vi "Draw Filled Rect.vi"(8 "Limits":dbl[](array[numeric]), 9 "Vision Instrumentation":T1, 10 "Target Data":T2={"Bounds"={"Left"=0.0, "Top"=0.0, "Right"=0.0, "Bottom"=0.0}, "Scores"={"Rect Coverage"=76.0, "Aspect Ratio"=0.0, "X Edge Strength"=40.0, "Y Edge Strength"=50.0}, "Clipped Edge"={"Left"=FALSE, "Top"=FALSE, "Right"=FALSE, "Bottom"=FALSE}}, 11 "image in":T3) -> (3 "image out":T3)   [LabVIEW 2011]
doc: "Add a rectangle border around the inside and outside of what is believed to be the reflective tape. Also place the color coded scores next to all of the large blobs being processed."
uses:
  <vilib>/vision/Image Controls.llb/IMAQ Image.ctl
  Target Data.ctl
  Vision Instrumentation Control.ctl
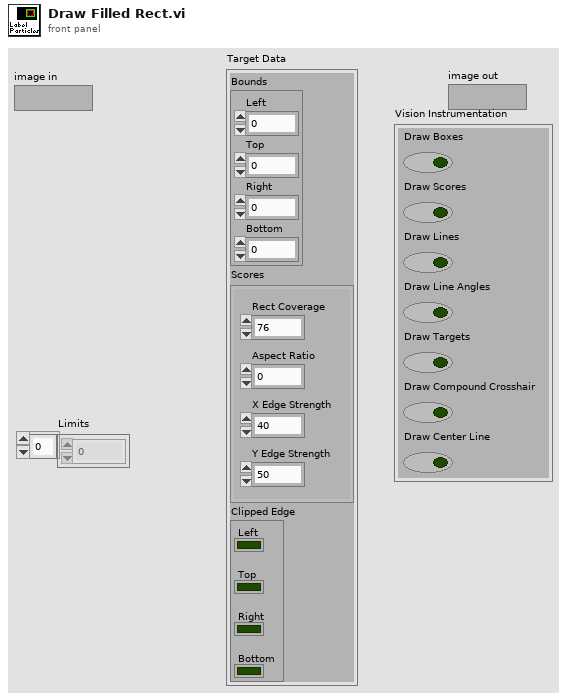
[diagram p1: front panel]
types:
  T1 = typedef "Vision Instrumentation Control.ctl" = cluster{"Draw Boxes":bool, "Draw Scores":bool, "Draw Lines":bool, "Draw Line Angles":bool, "Draw Targets":bool, "Draw Compound Crosshair":bool, "Draw Center Line":bool}
  T2 = typedef "Target Data.ctl" = cluster{"Bounds":cluster{"Left":dbl, "Top":dbl, "Right":dbl, "Bottom":dbl}, "Scores":cluster{"Rect Coverage":dbl, "Aspect Ratio":dbl, "X Edge Strength":dbl, "Y Edge Strength":dbl}, "Clipped Edge":cluster{"Left":bool, "Top":bool, "Right":bool, "Bottom":bool}}
  T3 = typedef "IMAQ Image.ctl" = refnum<image>
  T4 = cluster{"Left":dbl, "Top":dbl, "Right":dbl, "Bottom":dbl}
  T5 = cluster{"Rect Coverage":dbl, "Aspect Ratio":dbl, "X Edge Strength":dbl, "Y Edge Strength":dbl}
  T6 = cluster{"Left":bool, "Top":bool, "Right":bool, "Bottom":bool}
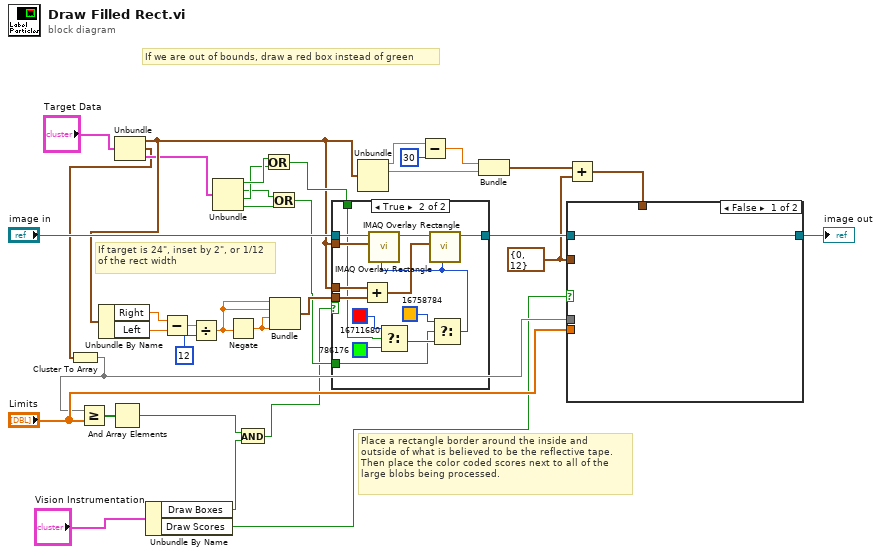
[diagram p0: block diagram]
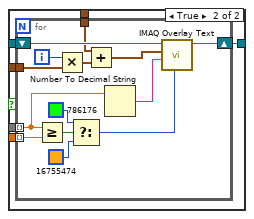
[diagram p2: hidden frame]
diagram:
  w24 = cluster{i32, i32} {0, 12}
  # "If we are out of bounds, draw a red box instead of green"
  # "Place a rectangle border around the inside and\noutside of what is believed to be the reflective tape.\nThen place the color coded scores next to all of the\nlarge blobs being processed."
  # "If target is 24\", inset by 2\", or 1/12\nof the rect width"
  n1 = Unbundle("Target Data") -> ("Bounds"=w9:T4, "Scores"=w6:T5, "Clipped Edge"=w7:T6)
  n2 = Cluster To Array(cluster=w6) -> (array=w8:dbl[])
  n3 = Greater Or Equal?(x=w8, y="Limits") -> (x >= y?=w33:bool[])
  n4 = Unbundle By Name(w9) -> ("Right"=w22:dbl, "Left"=w21:dbl)
  n5 = And Array Elements(Boolean array=w33) -> (logical AND=w3:bool)
  n6 = Unbundle By Name("Vision Instrumentation") -> ("Draw Boxes"=w4:bool, "Draw Scores"=w1:bool)
  n7 = Subtract(x=w22, y=w21) -> (x-y=w19:dbl)
  n8 = Divide(x=w19, y=12) -> (x/y=w17:dbl)
  n9 = Unbundle(w7) -> ("Left"=w16:bool, "Top"=w13:bool, "Right"=w15:bool, "Bottom"=w12:bool)
  n10 = Negate(x=w17) -> (-x=w23:dbl)
  n11 = And(x=w3, y=w4) -> (x .and. y?=w2:bool)
  n12 = Or(x=w16, y=w15) -> (x .or. y?=w14:bool)
  n13 = Or(x=w13, y=w12) -> (x .or. y?=w11:bool)
  n14 = Bundle(w17, w17, w23, w23) -> (w20:cluster{dbl, dbl, dbl, dbl})  [unwired: 1 in]
  n15 = case shown="True" w2 {
    tunnel: "image in" -> [w36 w50]
    tunnel: w9 -> [_ w49]
    tunnel: w9 -> [_ w47]
    tunnel: [w36 w45] -> w31
    tunnel: w20 -> [_ w44]
    tunnel: w14 -> [_ w38]
    tunnel: w11 -> [_ w37]
    frame False {
    }
    frame True {
      n16 = Add(x=w47, y=w44) -> (x+y=w46:cluster{dbl, dbl, dbl, dbl})
      n17 = Select(t=u32 16711680 ("Color"), s=w38, f=u32 786176 ("Color")) -> (s? t:f=w39:u32)
      n18 = Select(t=u32 16758784 ("Color"), s=w37, f=w39) -> (s? t:f=w40:u32)
      n19 = call "IMAQ Overlay Rectangle"("Color"=w40, "Rectangle"=w49, "Image"=w50) -> ("Image Out"=w48:T3)  [unwired: 3 in, 5 out]
      n20 = call "IMAQ Overlay Rectangle"("Color"=w40, "Rectangle"=w46, "Image"=w48) -> ("Image Out"=w45:T3)  [unwired: 3 in, 5 out]
    }
  }
  n21 = Unbundle(w9) -> ("Left"=w29:dbl, "Top"=w30:dbl)  [unwired: 2 out]
  n22 = Subtract(x=w29, y=30) -> (x-y=w28:dbl)
  n23 = Bundle(w28, "Top"=w30) -> (w26:cluster{dbl, "Top":dbl})  [unwired: 1 in]
  n24 = Add(x=w26, y=w24) -> (x+y=w25:cluster{dbl, dbl})
  n25 = case shown="False" w1 {
    tunnel: [w51 w57] -> w34
    tunnel: "Limits" -> [_ w56]
    tunnel: w31 -> [w51 w55]
    tunnel: w25 -> [_ w54]
    tunnel: w24 -> [_ w53]
    tunnel: w8 -> [_ w52]
    frame False {
    }
    frame True {
      n26 = for {
        shift-right: [w70] -> w57
        shift-left: w55 -> [w71]
        tunnel: w52 -> [w63] mode=indexing
        tunnel: w56 -> [w69] mode=indexing
        tunnel: w53 -> [w60]
        tunnel: w54 -> [w59]
        i -> [w62]
        n27 = Greater Or Equal?(x=w63, y=w69) -> (x >= y?=w68:bool)
        n28 = Multiply(x=w62, y=w60) -> (x*y=w61:cluster{i32, i32})
        n29 = Select(t=u32 786176 ("Color"), s=w68, f=u32 16755474 ("Color")) -> (s? t:f=w64:u32)
        n30 = Add(x=w59, y=w61) -> (x+y=w58:cluster{dbl, dbl})
        n31 = Number To Decimal String(number=w63) -> (decimal integer string=w65:string)  [unwired: 1 in]
        n32 = call "IMAQ Overlay Text"("Text Color (black)"=w64, "String"=w65, "Origin"=w58, "Image"=w71) -> ("Image Out"=w70:T3)  [unwired: 6 in, 1 out]
      }
    }
  }
  "image out" <- w34
